vi "Close Door.vi"(8 "error in (no error)":errorcluster, 11 "Doors Closed in":refnum<class "Doors Closed.lvclass">) -> (0 "error out":errorcluster, 3 "Doors Closed out":refnum<class "Doors Closed.lvclass">)   [LabVIEW 2020, in "Door Controller.lvlib" / "Doors Closed.lvclass"]
uses:
  Doors Closed.lvclass
  Door Controller/Door Controller.lvclass
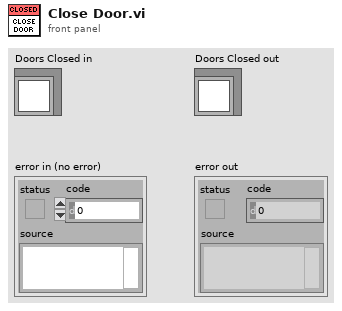
[diagram p1: front panel]
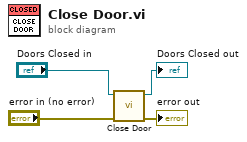
[diagram p0: block diagram]
diagram:
  n1 = call-parent "Close Door.vi"("error in (no error)"="error in (no error)", "Door Controller in"="Doors Closed in") -> ("error out"=→"error out":errorcluster, "Door Controller out"=→"Doors Closed out":refnum<class "Doors Closed.lvclass">)  [unwired: 8 in]
